vi "AlazarBeforeAsyncRead.vi"(6 "Flags":u32, 8 "error in (no error)":errorcluster, 9 "ASync Read Parameters [In]":T1, 10 "Channel Select":u32(ring)=1 items=["A"=1, "B"=2, "A + B"=3, "C"=4, "A + C"=5, "A + B"=6, "D"=8, "A + D"=9, "B + D"=10, "C + D"=12, "A + B + C + D"=15], 11 "Handle":u32) -> (0 "error out":errorcluster, 1 "ASync Read Parameters [Out]":T1, 2 "Return Code":u32, 3 "Handle":u32)   [LabVIEW 2018]
doc: "Configure a board to make an asynchronous AutoDMA acquisition."
uses:
  Controls/Async Read Parameters.ctl
  ATSApi.dll
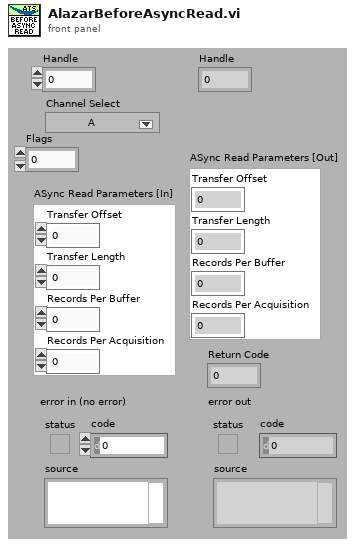
[diagram p1: front panel]
types:
  T1 = typedef "Async Read Parameters.ctl" = cluster{"Transfer Offset":u32, "Transfer Length":u32, "Records Per Buffer":u32, "Records Per Acquisition":u32}
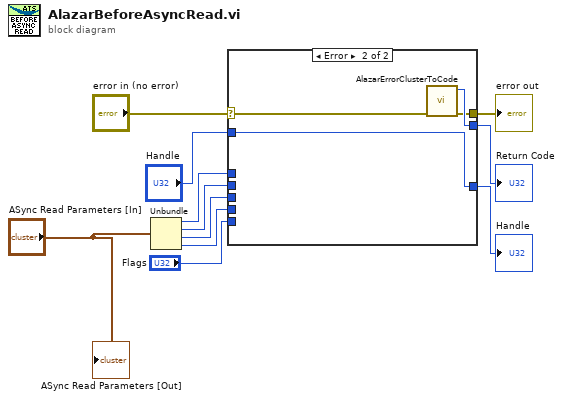
[diagram p0: block diagram]
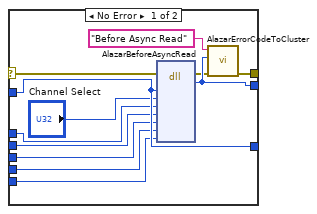
[diagram p2: hidden frame]
diagram:
  n1 = Unbundle("ASync Read Parameters [In]") -> ("Transfer Offset"=w5:u32, "Transfer Length"=w4:u32, "Records Per Buffer"=w3:u32, "Records Per Acquisition"=w2:u32)
  n2 = case shown="Error" "error in (no error)" {
    selector: "error in (no error)" -> [w12 w27]
    tunnel: [w21 w24] -> w10
    tunnel: [w23 w26] -> w9
    tunnel: "Handle" -> [w20 w25]
    tunnel: [w20 w25] -> w7
    tunnel: w5 -> [w18 _]
    tunnel: w4 -> [w17 _]
    tunnel: w3 -> [w16 _]
    tunnel: w2 -> [w15 _]
    tunnel: "Flags" -> [w14 _]
    frame No Error {
      n3 = dll-call lib="ATSApi.dll" fn="AlazarBeforeAsyncRead"(error in=w12, "handle"=w20, "channelSelect"="Channel Select", "transferOffset"=w18, "transferLength"=w17, "recordsPerBuffer"=w16, "recordsCount"=w15, "cFlags"=w14) -> (error out=w13:errorcluster, "return type"=w23:u32)  [unwired: 9 in, 1 out]
      n4 = call "AlazarErrorCodeToCluster.vi"("error in (no error)"=w13, "Error Code In"=w23, "Message"="Before Async Read") -> ("error out"=w21:errorcluster)  [unwired: 7 in, 1 out]
    }
    frame Error {
      n5 = call "AlazarErrorClusterToCode.vi"("error in (no error)"=w27) -> ("error out"=w24:errorcluster, "Error Code"=w26:u32)  [unwired: 9 in]
    }
  }
  "Handle" <- w7
  "error out" <- w10
  "Return Code" <- w9
  "ASync Read Parameters [Out]" <- "ASync Read Parameters [In]"
